vi "Configure Analog Alarm Type.vi"(0 "VISA resource name":refnum<visa-resource-name>, 1 "Unit Address (1)":u8=1 min=1 max=254, 5 "Alarm Number (1)":u16=1 min=1 max=4, 9 "Alarm Type (0: No Alarm)":u8(ring) items=["No Alarm", "Absolute High", "Absolute Low", "Deviation High", "Deviation Low", "Deviation Band", "Rising Rate of Change Alarm", "Falling Rate of Change Alarm"], 11 "error in (no error)":errorcluster) -> (4 "VISA resource name out":refnum<visa-resource-name>, 15 "error out":errorcluster)   [LabVIEW 2010, in "Eurotherm 32xx Series.lvlib"]
doc: "This VI configure analog alarm type.\nThe type of alarm determines when it will be triggered. Examples are a full scale high, where the input value has to be higher than the threshold to set the alarm off.\n\nWarning: This VI uses Controller Configuration Mode, this interrupts working process (device will not control).\nIt is recommended that the device should be disconnected from any active process."
uses:
  <instrlib>/Eurotherm 32xx Series/Eurotherm 32xx Series.lvlib
panel:
  # "The above shows graphically the operation of different types \nof alarm used in the controller. The graphs show changes \nin PV plotted against time. (Hysteresis set to zero)"
  # "PV"
  # "Full Scale High"
  # "Process Variable  (PV)"
  # "Deviation High"
  # "Setpoint (SP)"
  # "Deviation Low"
  # "Full Scale Low"
  # "Time"
  # "Full Scale Low"
  # "On"
  # "On"
  # "Deviation Low"
  # "On"
  # "On"
  # "Deviation High"
  # "On"
  # "Deviation Band"
  # "On"
  # "On"
  # "On"
  # "Full Scale High"
  # "On"
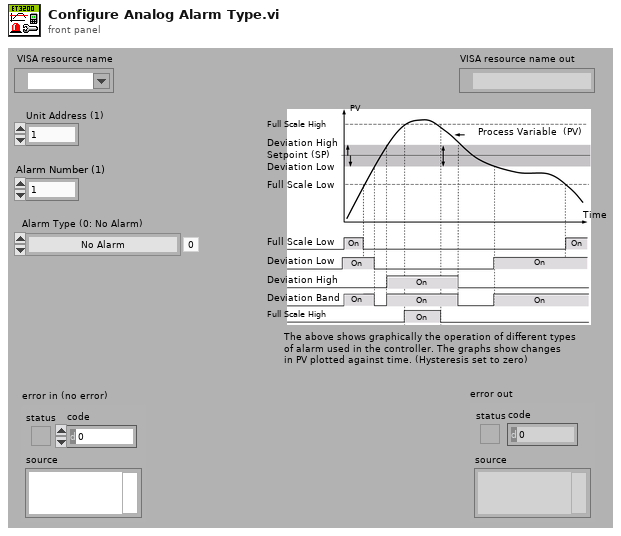
[diagram p1: front panel]
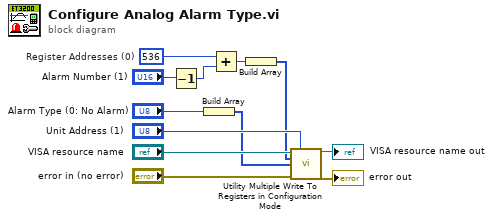
[diagram p0: block diagram]
diagram:
  w11 = u16 536  # Register Addresses (0)
  n1 = Decrement(x="Alarm Number (1)") -> (x-1=w1:u16)
  n2 = Build Array("Alarm Type (0: No Alarm)") -> (w4:u8[])
  n3 = Add(x=w11, y=w1) -> (x+y=w3:u16)
  n4 = Build Array(w3) -> (w2:u16[])
  n5 = call <instrlib>:"Utility Multiple Write To Registers in Configuration Mode.vi"("VISA resource name"="VISA resource name", "Unit Address (1)"="Unit Address (1)", "Registers Addresses (0)"=w2, "Data (0)"=w4, "error in (no error)"="error in (no error)") -> ("VISA resource name out"=→"VISA resource name out":refnum<visa-resource-name>, "error out"=→"error out":errorcluster)  [unwired: 9 in]
